vi "Implementation Example.vi"   [LabVIEW 2017]
uses:
  <vilib>/Rock Robotics/SystemInterfaces/DIO/FPGA_DIOPWMChannel.ctl
  <vilib>/Rock Robotics/WPI/SafetyOutput/WPI_SafetyOutputConfigMenu.ctl
  <vilib>/Rock Robotics/WPI/RobotDrive/WPI_RobotDriveOpen2MotorWithTalon.vi
  <vilib>/Rock Robotics/WPI/RobotDrive/WPI_RobotDriveArcadeDrive_Standard(NoSaturation).vi
  <vilib>/Rock Robotics/Network Tables/NT Write Numeric Array.vi
panel:
  # "Window -> Show Block Diagram for main code"
types:
  T1 = typedef "WPI_SafetyOutputConfigMenu.ctl" = enum16{"Enable", "Disable"}
  T2 = typedef "FPGA_DIOPWMChannel.ctl" = enum8{"PWM 0", "PWM 1", "PWM 2", "PWM 3", "PWM 4", "PWM 5", "PWM 6", "PWM 7", "PWM 8", "PWM 9", "PWM MXP 0", "PWM MXP 1", "PWM MXP 2", "PWM MXP 3", "PWM MXP 4", "PWM MXP 5", "PWM MXP 6", "PWM MXP 7", "PWM MXP 8", "PWM MXP 9", "Invalid"}
  T3 = typedef "WPI_RobotDriveDevRef.ctl" = cluster{"DevStatus":errorcluster, "Motors[]":T4[], "Square Inputs":bool, "Max Output":dbl}
  T4 = typedef "WPI_MotorControlDeviceRef.ctl" = cluster{"DeviceStatus":errorcluster, "Type":T5, "PWM":cluster{"PWM Channel":T2, "DeadBand":T6}, "CAN":cluster{"Device Number":u8, "SetOutput VI Ref":variant, "GetOutput VI Ref":variant, "Enable VI Ref":variant, "Disable VI Ref":variant, "Data":variant}, "Invert":bool, "DIO PWM":cluster{"PWM \"Enable\" Channel":T2, "DIOChannel":T7, "PWM Rate":dbl}}
  T5 = typedef "WPI_MotorControlType.ctl" = enum16{"PWM", "CAN", "DIO PWM"}
  T6 = typedef "WPI_PWMDeadband.ctl" = cluster{"Name":string, "maxPositivePwm":i32, "minPositivePwm":i32, "centerPwm":i32, "maxNegativePwm":i32, "minNegativePwm":i32, "angularRange":u16}
  T7 = typedef "FPGA_DIOChannel.ctl" = enum8{"DIO 0", "DIO 1", "DIO 2", "DIO 3", "DIO 4", "DIO 5", "DIO 6", "DIO 7", "DIO 8", "DIO 9", "DIO MXP 0", "DIO MXP 1", "DIO MXP 2", "DIO MXP 3", "DIO MXP 4", "DIO MXP 5", "DIO MXP 6", "DIO MXP 7", "DIO MXP 8", "DIO MXP 9", "DIO MXP 10", "DIO MXP 11", "DIO MXP 12", "DIO MXP 13", "DIO MXP 14", "DIO MXP 15", "SPI Port CS1", "SPI Port CS2", "SPI Port CS3", "SPI Port MISO", "SPI Port MOSI", "Invalid"}
  T8 = typedef "Command Status Info.ctl" = cluster{"Name":string, "Status":T9, "notifier out":T10}
  T9 = typedef "Completion Status.ctl" = enum16{"Successful", "Aborted", "Incomplete"}
  T10 = typedef "Completion Notifier.ctl" = refnum<notifier>
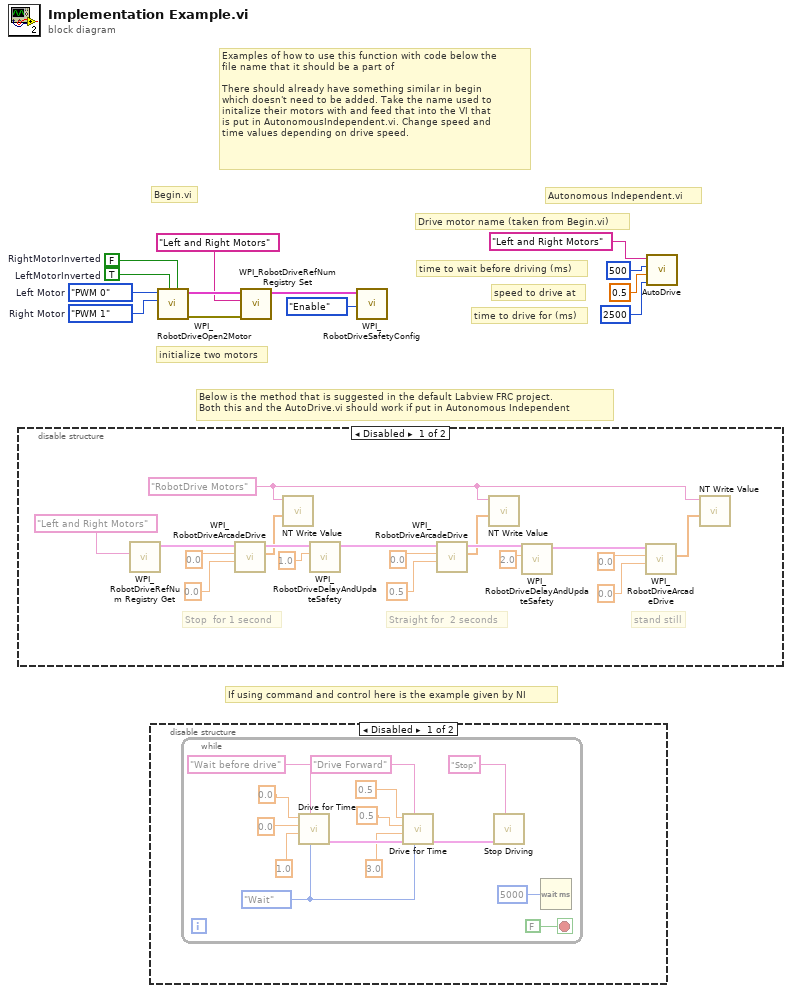
[diagram p0: block diagram]
diagram:
  w7 = FPGA_DIOPWMChannel."PWM 1"  # Right Motor
  w8 = FPGA_DIOPWMChannel."PWM 0"  # Left Motor
  w12 = TRUE  # LeftMotorInverted
  w13 = FALSE  # RightMotorInverted
  # "If using command and control here is the example given by NI"
  # "Below is the method that is suggested in the default Labview FRC project.\nBoth this and the AutoDrive.vi should work if put in Autonomous Independent"
  # "Examples of how to use this function with code below the \nfile name that it should be a part of\n\nThere should already have something similar in begin\nwhich doesn't need to be added. Take the name used to \ninitalize their motors with and feed that into the VI that \nis put in AutonomousIndependent.vi. Change speed and \ntime values depending on drive speed."
  # "time to drive for (ms)"
  # "speed to drive at"
  # "time to wait before driving (ms)"
  # "Drive motor name (taken from Begin.vi)"
  # "initialize two motors"
  # "Autonomous Independent.vi"
  # "Begin.vi"
  n1 = disable-structure shown="Disabled" {
    frame Disabled {
      w15 = "RobotDrive Motors" ("Name")
      # "stand still"
      # "Straight for  2 seconds"
      # "Stop  for 1 second"
      n2 = call <vilib>:"WPI_RobotDriveRefNum Registry Get.vi"("refnum name"="Left and Right Motors") -> ("RobotDriveDevRef"=w31:T3)  [unwired: 1 in, 9 out]
      n3 = call-poly <vilib>:"WPI_RobotDriveArcadeDrive.vi"("Y axis value"=0.0 ("X axis value"), "X axis value"=0.0, "RobotDriveDevRef"=w31) -> ("Motor Values"=w14:dbl[], "RobotDriveDevRef"=w24:T3)  [unwired: 1 in, 6 out]
      n4 = call-poly <vilib>:"NT Write Value.vi"("Numeric Array"=w14, "Name"=w15) -> ()  [unwired: 9 in, 1 out]
      n5 = call <vilib>:"WPI_RobotDriveDelayAndUpdateSafety.vi"("Delay (s)"=1.0, "RobotDriveDevRef"=w24) -> ("RobotDriveDevRef 2"=w25:T3)  [unwired: 8 in, 1 out]
      n6 = call-poly <vilib>:"WPI_RobotDriveArcadeDrive.vi"("Y axis value"=0.5 ("X axis value"), "X axis value"=0.0, "RobotDriveDevRef"=w25) -> ("Motor Values"=w16:dbl[], "RobotDriveDevRef"=w26:T3)  [unwired: 1 in, 6 out]
      n7 = call-poly <vilib>:"NT Write Value.vi"("Numeric Array"=w16, "Name"=w15) -> ()  [unwired: 9 in, 1 out]
      n8 = call <vilib>:"WPI_RobotDriveDelayAndUpdateSafety.vi"("Delay (s)"=2.0, "RobotDriveDevRef"=w26) -> ("RobotDriveDevRef 2"=w27:T3)  [unwired: 8 in, 1 out]
      n9 = call-poly <vilib>:"WPI_RobotDriveArcadeDrive.vi"("Y axis value"=0.0 ("X axis value"), "X axis value"=0.0, "RobotDriveDevRef"=w27) -> ("Motor Values"=w17:dbl[])  [unwired: 1 in, 7 out]
      n10 = call-poly <vilib>:"NT Write Value.vi"("Numeric Array"=w17, "Name"=w15) -> ()  [unwired: 9 in, 1 out]
    }
    frame Enabled {
    }
  }
  n11 = disable-structure shown="Disabled" {
    frame Disabled {
      n12 = while {
        stop <- FALSE stop-if-true
        w36 = enum16{"Start", "Wait"}."Wait" ("Synchronication")
        n13 = call "Drive for Time.vi"("Synchronization"=w36, "Description"="Wait before drive", "Seconds"=1.0 ("Delay (s)"), "Right Speed"=0.0 ("X axis value"), "Left Speed"=0.0 ("X axis value")) -> ("Command Info Out"=w45:T8)  [unwired: 5 in, 1 out]
        n14 = call "Drive for Time.vi"("Synchronization"=w36, "Description"="Drive Forward", "Command Info In"=w45, "Seconds"=3.0 ("Delay (s)"), "Right Speed"=0.5 ("X axis value"), "Left Speed"=0.5 ("X axis value")) -> ("Command Info Out"=w35:T8)  [unwired: 4 in, 1 out]
        n15 = call "Stop Driving.vi"("Description"="Stop", "Command Info In"=w35) -> ()  [unwired: 9 in, 1 out]
        n16 = Wait (ms)(milliseconds to wait=u32 5000 ("millisecond timer value")) -> ()  [unwired: 1 out]
      }
    }
    frame Enabled {
    }
  }
  n17 = call-poly <vilib>:"WPI_RobotDriveOpen2Motor.vi"("Right Motor Inverted"=w13, "Left Motor Inverted"=w12, "Right Motor"=w7, "Left Motor"=w8) -> ("error out"=w9:errorcluster, "RobotDriveDevRef"=w11:T3)  [unwired: 1 in, 5 out]
  n18 = call <vilib>:"WPI_RobotDriveRefNum Registry Set.vi"("error in (no error)"=w9, "refnum name"="Left and Right Motors", "RobotDriveDevRef"=w11) -> ("RobotDriveDevRef"=w6:T3)  [unwired: 1 in, 7 out]
  n19 = call <vilib>:"WPI_RobotDriveSafetyConfig.vi"("mode"=WPI_SafetyOutputConfigMenu."Enable", "RobotDriveDevRef"=w6) -> ()  [unwired: 8 in, 2 out]
  n20 = call "AutoDrive.vi"("Drive Time"=u32 2500, "Drive Speed"=0.5, "Wait before drive"=u32 500, "Motor Name"="Left and Right Motors") -> ()  [unwired: 8 in]
